vi "Collect.vi"(8 "error in (no error)":errorcluster, 11 "LabVIEW Collector in":refnum<class "LabVIEW Collector.lvclass">) -> (0 "error out":errorcluster, 2 "Metrics":refnum<data-value>[](array[refnum]), 3 "LabVIEW Collector out":refnum<class "LabVIEW Collector.lvclass">)   [LabVIEW 2020]
uses:
  <vilib>/TheLabVIEWLab/PromVIEW/collector/generic collector/Default Collector.lvclass
  <vilib>/TheLabVIEWLab/PromVIEW/collector/LabVIEW collector/LabVIEW Collector.lvclass
  C:/Github-locals/PromVIEW/src/collector/generic collector/Default Collector.lvclass
  C:/Github-locals/PromVIEW/src/collector/collectable/Collectable.lvclass
  C:/Github-locals/PromVIEW/src/collector/LabVIEW collector/LabVIEW Collector.lvclass
  <vilib>/TheLabVIEWLab/PromVIEW/metrics/metric/Metric.lvclass
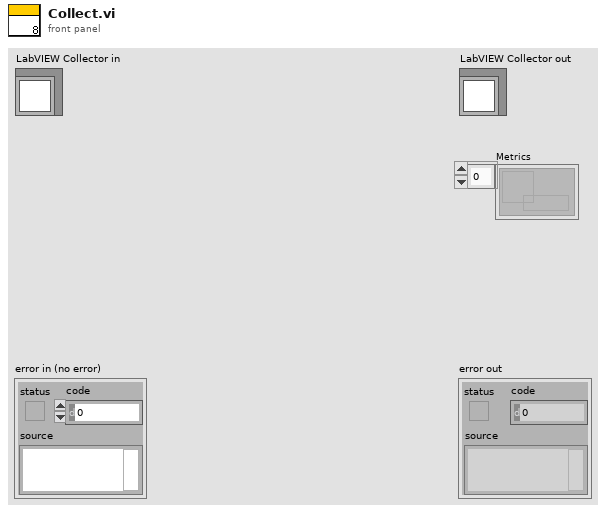
[diagram p1: front panel]
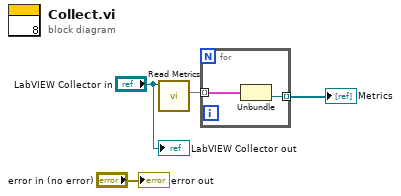
[diagram p0: block diagram]
diagram:
  n1 = call <vilib>:"Read Metrics.vi"("Default Collector in"="LabVIEW Collector in") -> ("Metrics"=w3:map{string, refnum<data-value>})  [unwired: 8 in, 2 out]
  n2 = for {
    tunnel: w3 -> [w6] mode=indexing
    tunnel: [w5] -> w2 mode=indexing
    n3 = Unbundle(w6) -> ("Metric"=w5:refnum<data-value>)  [unwired: 1 out]
  }
  "Metrics" <- w2
  "error out" <- "error in (no error)"
  "LabVIEW Collector out" <- "LabVIEW Collector in"
